vi "sub_Robot v1.vi"() -> ()   [LabVIEW 2017]
uses:
  <vilib>/Analysis/Matrix/Datatypes/RealMatrix.ctl
  Control/Force Torque Vector.ctl
  Control/State.ctl
  Control/Platform Vectors.ctl
  Control/Constants.ctl
  Control/Motor Position.ctl
  <vilib>/Analysis/baseanly.llb/A x Vector.vi
  <vilib>/DAQmx/read.llb/DAQmx Read (Analog 2D DBL NChan NSamp).vi
  <vilib>/Analysis/baseanly.llb/Mean (DBL).vi
  <vilib>/Analysis/baseanly.llb/Real A x B.vi
  <vilib>/Analysis/_algsub.llb/Vector Norm.vi
  <vilib>/Analysis/_algsub.llb/Real Vector Norm.vi
  <vilib>/Analysis/baseanly.llb/Outer Product.vi
  <vilib>/Analysis/baseanly.llb/Real Outer Product.vi
  <vilib>/robotics/Kinematics/Create Lie Group Matrix.vi
  <vilib>/Analysis/7linalg.llb/Create Special Real Matrix.vi
  <vilib>/Analysis/Matrix/Numeric/Multiply/Multiply.vi
  <vilib>/Analysis/Matrix/Numeric/Multiply/Multiply - RM,R.vi
  <vilib>/Analysis/Matrix/Numeric/Multiply/Multiply - R,RM.vi
  <vilib>/Analysis/Matrix/Numeric/Add/Add.vi
  <vilib>/Analysis/Matrix/Numeric/Add/Add - RM,RM.vi
  <vilib>/DAQmx/create/channels.llb/DAQmx Create Channel (AI-Voltage-Basic).vi
  <vilib>/DAQmx/configure/timing.llb/DAQmx Timing (Sample Clock).vi
  <vilib>/DAQmx/miscellaneous.llb/DAQmx Fill In Error Info.vi
  <vilib>/Analysis/3filter.llb/Butterworth Filter (DBL).vi
  <vilib>/Utility/inputDevices.llb/joystickAcquire.vi
  <vilib>/Analysis/NI_AALBase.lvlib
  <vilib>/robotics/Kinematics/NI_Kinematics.lvlib
  <vilib>/Analysis/NI_AALPro.lvlib
  <vilib>/Analysis/Matrix/NI_Matrix.lvlib
panel:
  in  "low cutoff freq: fl":dbl=0.1 format="%0.4f"
  in  "sampling freq: fs":dbl=100.0 format="%0.2f"
  in  "rate":dbl=1000.0 format="%#_13g"
  out "Motor Position":T1={"theta1"=1.8810837497796307, "theta2"=-0.7792215646198668, "theta3"=2.7030056815353944}
  in  "eta3":dbl=240.0
  in  "eta2":dbl=120.0
  in  "eta1":dbl
  out "dt":dbl=0.014741399998456473
  in  "gamma2":dbl=72.0
  in  "gamma1":dbl=90.0
  in  "alpha2":dbl=90.0
  in  "alpha1":dbl=90.0
  out "Constants":T2={"alpha1"=1.5707963267948966, "alpha2"=1.5707963267948966, "beta1"=0.9553166181245093, "beta2"=0.7460127831658564, "gamma1"=1.5707963267948966, "gamma2"=1.2566370614359172, "eta1"=0.0, "eta2"=2.0943951023931953, "eta3"=4.1887902047863905}
  out "Platform Vectors":T3={"v1"=[0.9518431395713998, -0.15246563731281282, 0.26598659193586577], "v2"=[0.43921969187034554, 0.8926089520236044, 0.10166278099993067], "v3"=[0.5741590303779587, 0.15523155866204005, -0.8038933828753619]}
  in  "radius":dbl=0.1
  in  "State":T4={"Inertia"=0.0, "Damping"=0.5, "RoM"=0.0}
  out "Waveform Chart":cluster{dbl, dbl, dbl}(graph)
  out "Force Torque Vector":T5
  in  "Calibration Matrix":T6=[[0.70287, 0.28046, -1.06379, -47.58271, -1.64459, 46.90249], [-0.12905, 55.12684, -1.23322, -27.09022, 0.94146, -27.44249], [69.23154, 1.17633, 67.18151, 0.05352, 69.14468, -0.82584], [0.02366, 0.38743, -1.10802, -0.19684, 1.1351, -0.20033], [1.26658, 0.02633, -0.60731, 0.32903, -0.6386, -0.32248], [0.02624, -0.70869, -0.00313, -0.69424, -0.02408, -0.68399]]
  in  "stop":bool
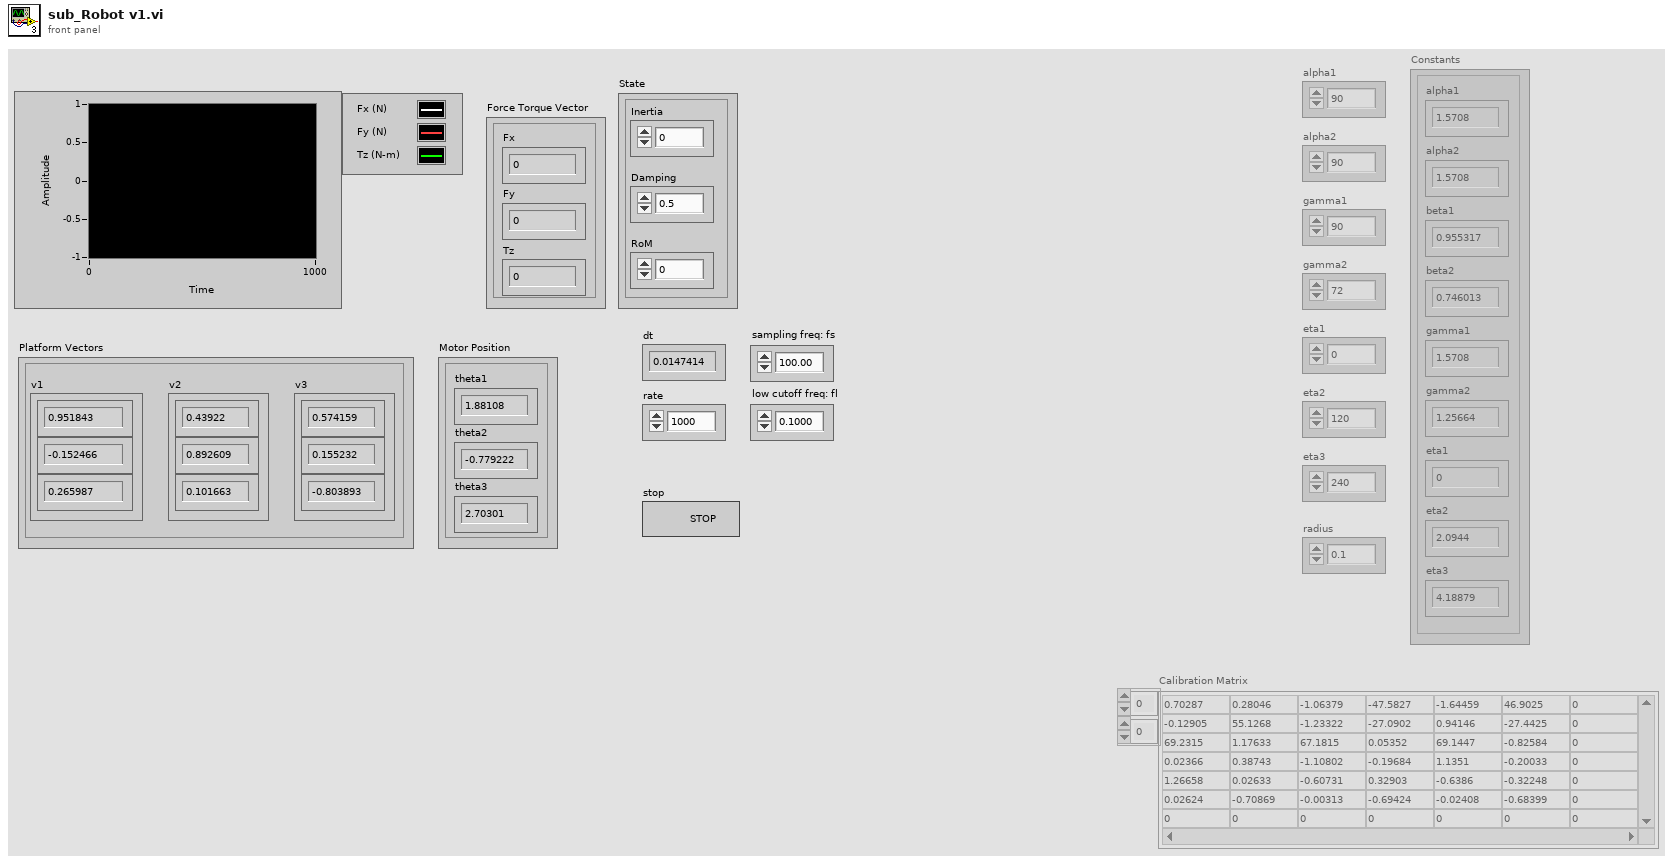
[diagram p1: front panel]
types:
  T1 = typedef "Motor Position.ctl" = cluster{"theta1":dbl, "theta2":dbl, "theta3":dbl}
  T2 = typedef "Constants.ctl" = cluster{"alpha1":dbl, "alpha2":dbl, "beta1":dbl, "beta2":dbl, "gamma1":dbl, "gamma2":dbl, "eta1":dbl, "eta2":dbl, "eta3":dbl}
  T3 = typedef "Platform Vectors.ctl" = cluster{"v1":dbl[], "v2":dbl[], "v3":dbl[]}
  T4 = typedef "State.ctl" = cluster{"Inertia":dbl, "Damping":dbl, "RoM":dbl}
  T5 = typedef "Force Torque Vector.ctl" = cluster{"Fx":dbl, "Fy":dbl, "Tz":dbl}
  T6 = typedef "NI_Matrix.lvlib/RealMatrix.ctl" = dbl[][]
  T7 = cluster{"X axis":i32, "Y axis":i32, "Z axis":i32, "X axis rotation":i32, "Y axis rotation":i32, "Z axis rotation":i32, "U axis":i32, "V axis":i32}
  T8 = cluster{"element":dbl, "element":dbl, "element":dbl}
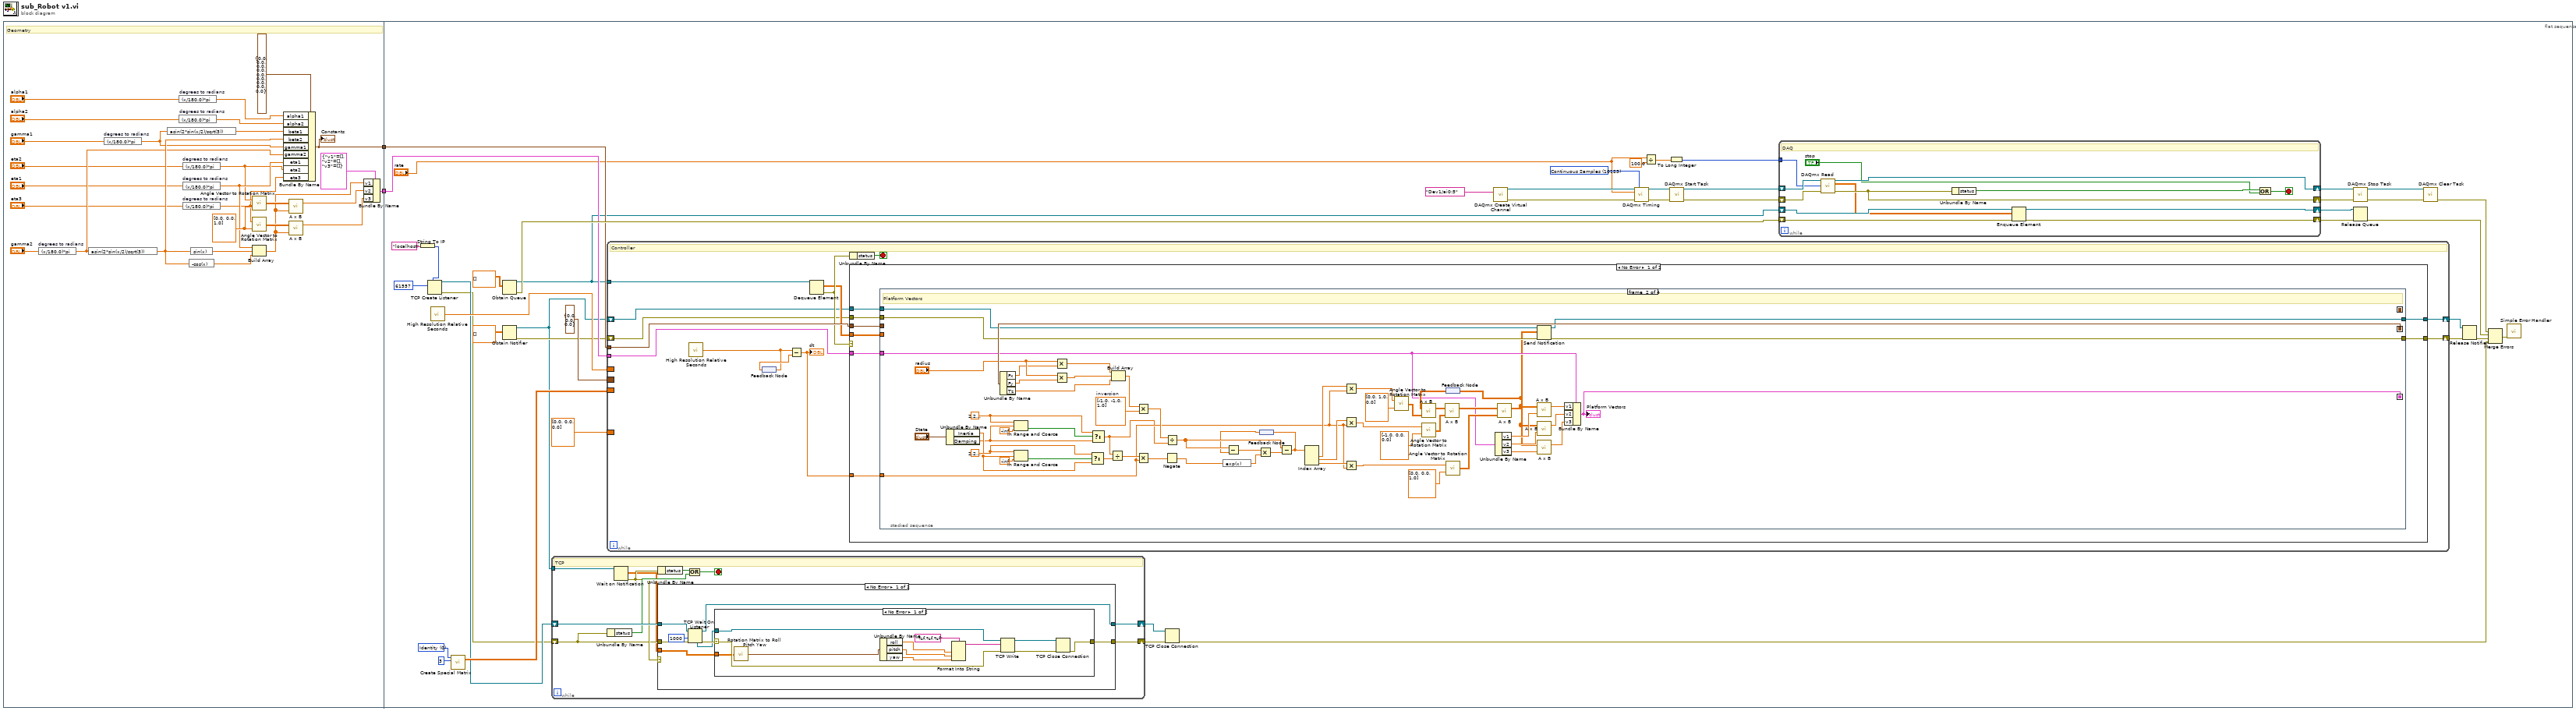
[diagram p0: block diagram]
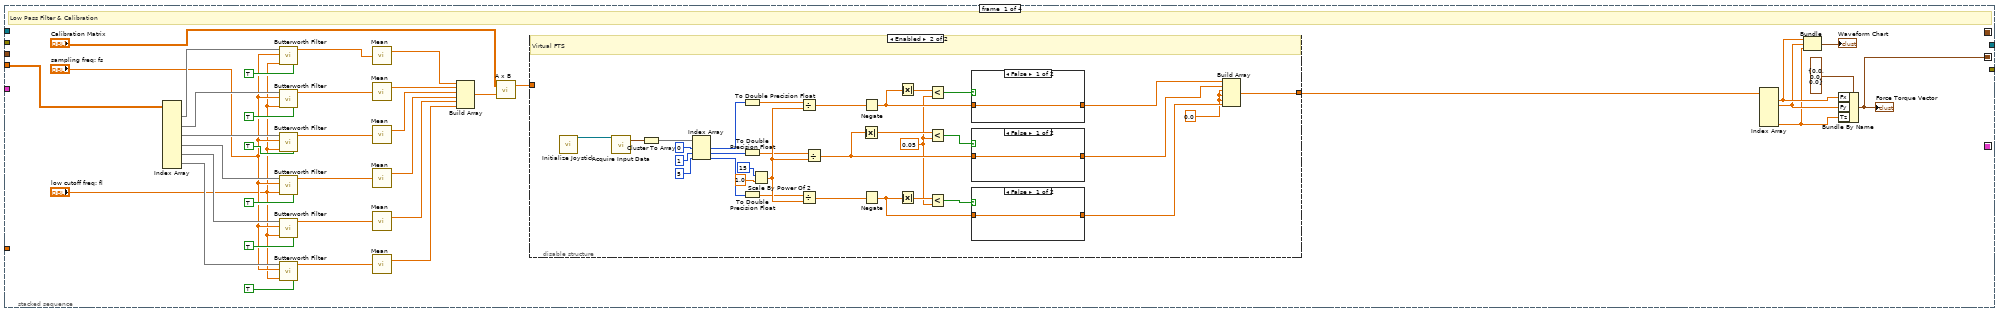
[diagram p4: hidden frame]
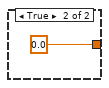
[diagram p6: hidden frame]
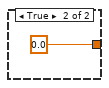
[diagram p7: hidden frame]
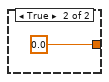
[diagram p8: hidden frame]
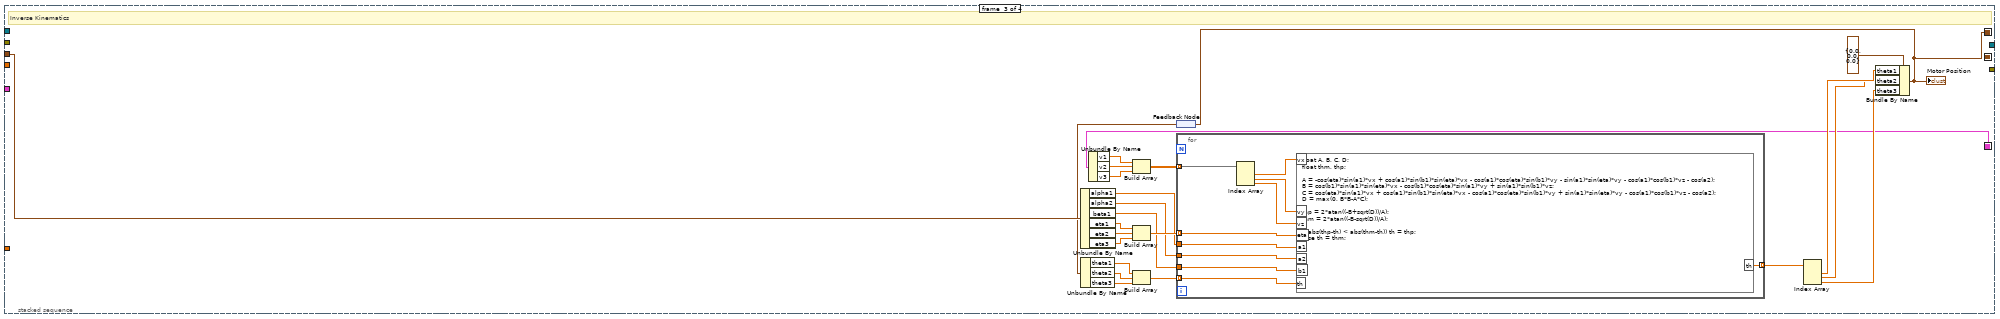
[diagram p9: hidden frame]
diagram:
  n1 = flat-sequence {
    tunnel: [w3] -> w2
    tunnel: [w5] -> w1
    tunnel: w2 -> [w54]
    tunnel: w1 -> [w53]
    frame #0 {
      w19 = dbl[] [0.0, 0.0, 1.0] ("vector")
      # "Geometry"
      n2 = expression code="(x/180.0)*pi" "degrees to radians"("gamma2") -> (w13:dbl)
      n3 = expression code="asin(2*sin(x/2)/sqrt(3))"(w13) -> (w15:dbl)
      n4 = expression code="(x/180.0)*pi" "degrees to radians"("gamma1") -> (w14:dbl)
      n5 = expression code="asin(2*sin(x/2)/sqrt(3))"(w14) -> (w26:dbl)
      n6 = expression code="(x/180.0)*pi" "degrees to radians"("alpha1") -> (w29:dbl)
      n7 = expression code="(x/180.0)*pi" "degrees to radians"("alpha2") -> (w27:dbl)
      n8 = expression code="(x/180.0)*pi" "degrees to radians"("eta2") -> (w8:dbl)
      n9 = expression code="(x/180.0)*pi" "degrees to radians"("eta1") -> (w9:dbl)
      n10 = expression code="(x/180.0)*pi" "degrees to radians"("eta3") -> (w7:dbl)
      n11 = expression code="-cos(x)"(w15) -> (w21:dbl)
      n12 = expression code="sin(x)"(w15) -> (w20:dbl)
      n13 = call <vilib>:"Angle Vector to Rotation Matrix.vi"("vector"=w19, "angle"=w8) -> ("rotation matrix"=w22:T6)
      n14 = call <vilib>:"Angle Vector to Rotation Matrix.vi"("vector"=w19, "angle"=w7) -> ("rotation matrix"=w23:T6)
      n15 = Build Array(w9, w20, w21) -> (w18:dbl[])
      n16 = Bundle By Name(cluster=T2 {"alpha1"=0.0, "alpha2"=0.0, "beta1"=0.0, "beta2"=0.0, "gamma1"=0.0, "gamma2"=0.0, "eta1"=0.0, "eta2"=0.0, "eta3"=0.0} ("Constants"), "alpha1"=w29, "alpha2"=w27, "beta1"=w26, "beta2"=w15, "gamma1"=w14, "gamma2"=w13, "eta1"=w9, "eta2"=w8, "eta3"=w7) -> (w5:T2)
      "Constants" <- w5
      n17 = call-poly <vilib>:"A x B.vi"("Vector"=w18, "A"=w22) -> ("A x Vector"=w17:dbl[])  [unwired: 1 out]
      n18 = call-poly <vilib>:"A x B.vi"("Vector"=w18, "A"=w23) -> ("A x Vector"=w16:dbl[])  [unwired: 1 out]
      n19 = Bundle By Name(cluster=T3 {"v1"=[], "v2"=[], "v3"=[]} ("Platform Vectors"), "v1"=w18, "v2"=w17, "v3"=w16) -> (w3:T3)
    }
    frame #1 {
      w57 = 0 items=["Identity", "Diagonal", "Toeplitz", "Vandermonde", "Companion", "Hankel", "Hadamard", "Wilkinson", "Hilbert", "Inverse Hilbert", "Rosser", "Pascal"] ("matrix type")
      w65 = 10123 items=["Finite Samples"=10178, "Continuous Samples"=10123, "Hardware Timed Single Point"=12522] ("sample mode")
      n20 = String To IP(1:"localhost" ("name")) -> (0:w33:u32)
      n21 = TCP Create Listener(7:w33, 10:u16 61557 ("port")) -> (0:w31:errorcluster, 3:w32:refnum<k5>)  [unwired: 3 in, 1 out]
      n22 = call <vilib>:"High Resolution Relative Seconds.vi"() -> ("relative seconds"=w46:dbl)
      n23 = call-poly <vilib>:"Create Special Matrix.vi"("matrix type"=w57, "matrix size"=3) -> ("Special Matrix"=w55:T6)  [unwired: 3 in, 1 out]
      n24 = Obtain Queue(element data type=dbl[][] [] ("data")) -> (queue out=w51:refnum<queue>, error out=w64:errorcluster)  [unwired: 4 in, 1 out]
      n25 = Obtain Notifier(notification data type=T6 [] ("A x B")) -> (notifier out=w40:refnum<notifier>, error out=w44:errorcluster)  [unwired: 3 in, 1 out]
      n26 = while {
        tunnel: w40 -> [w86]
        shift-right: [w84] -> w37
        shift-left: w31 -> [w79]
        shift-right: [w85] -> w38
        shift-left: w32 -> [w83]
        stop <- w78 stop-if-true
        # "TCP"
        n27 = Unbundle By Name(w79) -> ("status"=w81:bool)
        n28 = Wait on Notification(notifier=w86) -> (notification=w77:T6, error out=w80:errorcluster)  [unwired: 3 in, 2 out]
        n29 = Unbundle By Name(w80) -> ("status"=w82:bool)
        n30 = case shown="No Error" w80 {
          tunnel: w79 -> [w93 w108]
          tunnel: [w92 w109] -> w85
          tunnel: [w90 w108] -> w84
          tunnel: w83 -> [w89 w109]
          tunnel: w77 -> [w88 _]
          frame No Error {
            n31 = TCP Wait On Listener(8:w93, 9:1000 ("timeout ms (wait forever: -1)"), 11:w89) -> (0:w94:errorcluster, 3:w92:refnum<k5>, 4:w91:refnum<k5>)  [unwired: 1 in, 2 out]
            n32 = case shown="No Error" w94 {
              selector: w94 -> [w102 w107]
              tunnel: w91 -> [w105 _]
              tunnel: [w103 w107] -> w90
              tunnel: w88 -> [w96 _]
              frame No Error {
                n33 = call <vilib>:"Rotation Matrix to Roll Pitch Yaw.vi"("rotation matrix"=w96) -> ("angles"=w98:cluster{"roll":dbl, "pitch":dbl, "yaw":dbl})
                n34 = Unbundle By Name(w98) -> ("roll"=w99:dbl, "pitch"=w100:dbl, "yaw"=w101:dbl)
                n35 = Format Into String(format string="%f,%f,%f", w99, w100, w101) -> (resulting string=w95:string)  [unwired: 2 in, 1 out]
                n36 = TCP Write(connection ID=w105, data in=w95, error in (no error)=w102) -> (connection ID out=w106:refnum<k5>, error out=w104:errorcluster)  [unwired: 1 in, 1 out]
                n37 = TCP Close Connection(connection ID=w106, error in (no error)=w104) -> (error out=w103:errorcluster)  [unwired: 1 in, 1 out]
              }
              frame Error {
              }
            }
          }
          frame Error {
          }
        }
        n38 = Compound Arithmetic op=OR(w82, w81) -> (w78:bool)
      }
      n39 = while {
        tunnel: w51 -> [w122]
        border: dbl[] [0.0, 0.0, 0.0] -> [_]
        border: w55 -> [_]
        tunnel: w53 -> [w120]
        border: T1 {"theta1"=0.0, "theta2"=0.0, "theta3"=0.0} ("Motor Position") -> [_]
        border: w46 -> [_]
        tunnel: w54 -> [w121]
        shift-right: [w113] -> w43
        shift-left: w40 -> [w114]
        shift-right: [w111] -> w42
        shift-left: w44 -> [w112]
        stop <- w110 stop-if-true
        # "Controller"
        n40 = call <vilib>:"High Resolution Relative Seconds.vi"() -> ("relative seconds"=w116:dbl)
        n41 = feedback-in #1(w116) -> ()
        n42 = feedback #1() -> (w117:dbl)
        n43 = Subtract(x=w116, y=w117) -> (x-y=w115:dbl)
        "dt" <- w115
        n44 = Dequeue Element(queue=w122) -> (element=w118:dbl[][], error out=w119:errorcluster)  [unwired: 2 in, 2 out]
        n45 = Unbundle By Name(w119) -> ("status"=w110:bool)
        n46 = case shown="No Error" w119 {
          tunnel: w121 -> [w130 _]
          tunnel: w120 -> [w129 _]
          tunnel: w118 -> [w128 _]
          tunnel: w115 -> [w127 _]
          tunnel: w114 -> [w126 w301]
          tunnel: [w123 w301] -> w113
          tunnel: w112 -> [w125 w300]
          tunnel: [w124 w300] -> w111
          frame No Error {
            n47 = stacked-sequence {
              seq-local: [w165 _ _ _] -> [_ w244 _ _]
              seq-local: [_ w227 _ _] -> [_ _ w268 _]
              seq-local: [_ _ w266 _] -> [_ _ _ _]
              tunnel: w130 -> [_ w231 _ _]
              tunnel: w129 -> [_ _ w285 _]
              tunnel: w127 -> [_ w226 _ _]
              tunnel: w128 -> [w137 _ _ _]
              tunnel: w126 -> [_ w211 _ _]
              tunnel: w125 -> [_ w210 _ _]
              tunnel: [_ w209 _ _] -> w124
              tunnel: [_ w208 _ _] -> w123
              frame #0 {
                # "Low Pass Filter & Calibration"
                n48 = Index Array(array=w137) -> (element #1=w148:dbl[], element #2=w147:dbl[], element #3=w146:dbl[], element #4=w145:dbl[], element #5=w144:dbl[], element #6=w143:dbl[])  [unwired: 12 in]
                n49 = call-poly <vilib>:"Butterworth Filter.vi"("init/cont (init:F)"=TRUE, "low cutoff freq: fl"="low cutoff freq: fl", "sampling freq: fs"="sampling freq: fs", "X"=w148) -> ("Filtered X"=w149:dbl[])  [unwired: 4 in, 1 out]
                n50 = call-poly <vilib>:"Butterworth Filter.vi"("init/cont (init:F)"=TRUE, "low cutoff freq: fl"="low cutoff freq: fl", "sampling freq: fs"="sampling freq: fs", "X"=w147) -> ("Filtered X"=w151:dbl[])  [unwired: 4 in, 1 out]
                n51 = call-poly <vilib>:"Butterworth Filter.vi"("init/cont (init:F)"=TRUE, "low cutoff freq: fl"="low cutoff freq: fl", "sampling freq: fs"="sampling freq: fs", "X"=w146) -> ("Filtered X"=w153:dbl[])  [unwired: 4 in, 1 out]
                n52 = call-poly <vilib>:"Butterworth Filter.vi"("init/cont (init:F)"=TRUE, "low cutoff freq: fl"="low cutoff freq: fl", "sampling freq: fs"="sampling freq: fs", "X"=w145) -> ("Filtered X"=w154:dbl[])  [unwired: 4 in, 1 out]
                n53 = call-poly <vilib>:"Butterworth Filter.vi"("init/cont (init:F)"=TRUE, "low cutoff freq: fl"="low cutoff freq: fl", "sampling freq: fs"="sampling freq: fs", "X"=w144) -> ("Filtered X"=w155:dbl[])  [unwired: 4 in, 1 out]
                n54 = call-poly <vilib>:"Butterworth Filter.vi"("init/cont (init:F)"=TRUE, "low cutoff freq: fl"="low cutoff freq: fl", "sampling freq: fs"="sampling freq: fs", "X"=w143) -> ("Filtered X"=w159:dbl[])  [unwired: 4 in, 1 out]
                n55 = call-poly <vilib>:"Mean.vi"("X"=w149) -> ("mean"=w150:dbl)  [unwired: 1 out]
                n56 = call-poly <vilib>:"Mean.vi"("X"=w151) -> ("mean"=w152:dbl)  [unwired: 1 out]
                n57 = call-poly <vilib>:"Mean.vi"("X"=w153) -> ("mean"=w156:dbl)  [unwired: 1 out]
                n58 = call-poly <vilib>:"Mean.vi"("X"=w154) -> ("mean"=w157:dbl)  [unwired: 1 out]
                n59 = call-poly <vilib>:"Mean.vi"("X"=w155) -> ("mean"=w158:dbl)  [unwired: 1 out]
                n60 = call-poly <vilib>:"Mean.vi"("X"=w159) -> ("mean"=w160:dbl)  [unwired: 1 out]
                n61 = Build Array(w150, w152, w156, w157, w158, w160) -> (w135:dbl[])
                n62 = call-poly <vilib>:"A x B.vi"("Vector"=w135, "A"="Calibration Matrix") -> ("A x Vector"=w131:dbl[])  [unwired: 1 out]
                n63 = disable-structure shown="Enabled" {
                  disable-tunnel: [w168 w176] -> w132
                  disable-tunnel: w131 -> [w168 _]
                  frame Disabled {
                  }
                  frame Enabled {
                    w175 = 0.0 ("element")
                    w180 = 0.05 ("y")
                    # "Virtual FTS"
                    n64 = call <vilib>:"Initialize Joystick.vi"() -> ("device ID"=w193:refnum<k1>)  [unwired: 10 in, 1 out]
                    n65 = call-poly <vilib>:"Acquire Input Data.vi"("device ID"=w193) -> ("axis info"=w200:T7)  [unwired: 14 in, 4 out]
                    n66 = Cluster To Array(cluster=w200) -> (array=w196:i32[])
                    n67 = Index Array(array=w196, index #1=0 ("index"), index #2=1 ("index"), index #3=5 ("index")) -> (element #1=w174:i32, element #2=w172:i32, element #3=w170:i32)
                    n68 = To Double Precision Float(number=w174) -> (double precision float=w173:dbl)
                    n69 = To Double Precision Float(number=w172) -> (double precision float=w171:dbl)
                    n70 = To Double Precision Float(number=w170) -> (double precision float=w169:dbl)
                    n71 = Scale By Power Of 2(n=i16 15, x=1.0) -> (x*2^n=w188:dbl)
                    n72 = Divide(x=w173, y=w188) -> (x/y=w192:dbl)
                    n73 = Divide(x=w169, y=w188) -> (x/y=w181:dbl)
                    n74 = Divide(x=w171, y=w188) -> (x/y=w183:dbl)
                    n75 = Absolute Value(x=w183) -> (abs(x)=w190:dbl)
                    n76 = Negate(x=w192) -> (-x=w184:dbl)
                    n77 = Negate(x=w181) -> (-x=w182:dbl)
                    n78 = Absolute Value(x=w184) -> (abs(x)=w191:dbl)
                    n79 = Absolute Value(x=w182) -> (abs(x)=w189:dbl)
                    n80 = Less?(x=w191, y=w180) -> (x < y?=w187:bool)
                    n81 = Less?(x=w190, y=w180) -> (x < y?=w186:bool)
                    n82 = Less?(x=w189, y=w180) -> (x < y?=w185:bool)
                    n83 = case shown="False" w187 {
                      tunnel: [w205 0.0] -> w179
                      tunnel: w184 -> [w205 _]
                      frame False {
                      }
                      frame True {
                      }
                    }
                    n84 = case shown="False" w186 {
                      tunnel: [w203 0.0] -> w178
                      tunnel: w183 -> [w203 _]
                      frame False {
                      }
                      frame True {
                      }
                    }
                    n85 = case shown="False" w185 {
                      tunnel: [w201 0.0] -> w177
                      tunnel: w182 -> [w201 _]
                      frame False {
                      }
                      frame True {
                      }
                    }
                    n86 = Build Array(w179, w178, w175, w175, w175, w177) -> (w176:dbl[])
                  }
                }
                n87 = Index Array(array=w132) -> (element #1=w164:dbl, element #2=w163:dbl, element #6=w162:dbl)  [unwired: 6 in, 3 out]
                n88 = Bundle("element"=w164, "element"=w163, "element"=w162) -> (→"Waveform Chart":T8)  [unwired: 1 in]
                n89 = Bundle By Name(cluster=T5 {"Fx"=0.0, "Fy"=0.0, "Tz"=0.0} ("Force Torque Vector"), "Fx"=w164, "Fy"=w163, "Tz"=w162) -> (w165:T5)
                "Force Torque Vector" <- w165
              }
              frame #1 {
                w216 = 2.220446049250313e-16
                w219 = 2.220446049250313e-16
                w229 = dbl[] [-1.0, -1.0, 1.0]  # inversion
                # "Platform Vectors"
                n90 = Unbundle By Name("State") -> ("Inertia"=w218:dbl, "Damping"=w213:dbl)
                n91 = Unbundle By Name(w244) -> ("Fx"=w242:dbl, "Fy"=w241:dbl, "Tz"=w238:dbl)
                n92 = In Range and Coerce(upper limit=w216, x=w213, lower limit=-inf) -> (In Range?=w215:bool)  [unwired: 1 out]
                n93 = In Range and Coerce(upper limit=w219, x=w218, lower limit=-inf) -> (In Range?=w220:bool)  [unwired: 1 out]
                n94 = Multiply(x="radius", y=w242) -> (x*y=w240:dbl)
                n95 = Multiply(x="radius", y=w241) -> (x*y=w239:dbl)
                n96 = Select(t=w219, s=w220, f=w218) -> (s? t:f=w217:dbl)
                n97 = Select(t=w216, s=w215, f=w213) -> (s? t:f=w212:dbl)
                n98 = Divide(x=w212, y=w217) -> (x/y=w255:dbl)
                n99 = Build Array(w240, w239, w238) -> (w230:dbl[])
                n100 = Multiply(x=w230, y=w229) -> (x*y=w228:dbl[])
                n101 = Multiply(x=w255, y=w226) -> (x*y=w254:dbl)
                n102 = Negate(x=w254) -> (-x=w253:dbl)
                n103 = Divide(x=w228, y=w212) -> (x/y=w250:dbl[])
                n104 = expression code="exp(x)"(w253) -> (w251:dbl)
                n105 = feedback #2() -> (w236:dbl[])
                n106 = Subtract(x=w250, y=w236) -> (x-y=w252:dbl[])
                n107 = Multiply(x=w252, y=w251) -> (x*y=w249:dbl[])
                n108 = Subtract(x=w250, y=w249) -> (x-y=w237:dbl[])
                n109 = feedback-in #2(w237) -> ()
                n110 = Index Array(array=w237) -> (element #1=w247:dbl, element #2=w246:dbl, element #3=w248:dbl)  [unwired: 3 in]
                n111 = Multiply(x=w247, y=w226) -> (x*y=w265:dbl)
                n112 = Multiply(x=w246, y=w226) -> (x*y=w264:dbl)
                n113 = Multiply(x=w248, y=w226) -> (x*y=w225:dbl)
                n114 = call <vilib>:"Angle Vector to Rotation Matrix.vi"("vector"=dbl[] [0.0, 1.0, 0.0], "angle"=w265) -> ("rotation matrix"=w260:T6)
                n115 = call <vilib>:"Angle Vector to Rotation Matrix.vi"("vector"=dbl[] [-1.0, 0.0, 0.0], "angle"=w264) -> ("rotation matrix"=w258:T6)
                n116 = feedback #3() -> (w235:T6)
                n117 = call-poly <vilib>:"A x B.vi"("B"=w260, "A"=w235) -> ("A x B"=w259:T6)  [unwired: 1 out]
                n118 = call-poly <vilib>:"A x B.vi"("B"=w258, "A"=w259) -> ("A x B"=w257:T6)  [unwired: 1 out]
                n119 = call <vilib>:"Angle Vector to Rotation Matrix.vi"("vector"=dbl[] [0.0, 0.0, 1.0], "angle"=w225) -> ("rotation matrix"=w256:T6)
                n120 = Unbundle By Name(w231) -> ("v1"=w234:dbl[], "v2"=w233:dbl[], "v3"=w232:dbl[])
                n121 = call-poly <vilib>:"A x B.vi"("B"=w256, "A"=w257) -> ("A x B"=w207:T6)  [unwired: 1 out]
                n122 = feedback-in #3(w207) -> ()
                n123 = Send Notification(notification=w207, notifier=w211, error in (no error)=w210) -> (notifier out=w208:refnum<notifier>, error out=w209:errorcluster)
                n124 = call-poly <vilib>:"A x B.vi"("Vector"=w234, "A"=w207) -> ("A x Vector"=w224:dbl[])  [unwired: 1 out]
                n125 = call-poly <vilib>:"A x B.vi"("Vector"=w233, "A"=w207) -> ("A x Vector"=w223:dbl[])  [unwired: 1 out]
                n126 = call-poly <vilib>:"A x B.vi"("Vector"=w232, "A"=w207) -> ("A x Vector"=w222:dbl[])  [unwired: 1 out]
                n127 = Bundle By Name(cluster=w231, "v1"=w224, "v2"=w223, "v3"=w222) -> (w227:T3)
                "Platform Vectors" <- w227
              }
              frame #2 {
                # "Inverse Kinematics"
                n128 = Unbundle By Name(w285) -> ("alpha1"=w280:dbl, "alpha2"=w279:dbl, "beta1"=w278:dbl, "eta1"=w284:dbl, "eta2"=w283:dbl, "eta3"=w282:dbl)
                n129 = Unbundle By Name(w268) -> ("v1"=w289:dbl[], "v2"=w288:dbl[], "v3"=w287:dbl[])
                n130 = Build Array(w289, w288, w287) -> (w286:dbl[][])
                n131 = Build Array(w284, w283, w282) -> (w281:dbl[])
                n132 = feedback #4() -> (w273:T1)
                n133 = Unbundle By Name(w273) -> ("theta1"=w272:dbl, "theta2"=w271:dbl, "theta3"=w270:dbl)
                n134 = Build Array(w272, w271, w270) -> (w269:dbl[])
                n135 = for {
                  tunnel: w286 -> [w299] mode=indexing
                  tunnel: w281 -> [w295] mode=indexing
                  tunnel: w280 -> [w294]
                  tunnel: w279 -> [w293]
                  tunnel: w278 -> [w292]
                  tunnel: [w291] -> w277 mode=indexing
                  tunnel: w269 -> [w290] mode=indexing
                  n136 = Index Array(array=w299) -> (element #1=w298:dbl, element #2=w297:dbl, element #3=w296:dbl)  [unwired: 3 in]
                  n137 = formula code="float A, B, C, D;\nfloat thm, thp;\n\nA = -cos(eta)*sin(a1)*vx + cos(a1)*sin(b1)*sin(eta)*vx - cos(a1)*cos(eta)*sin(b1)*vy - sin(a1)*sin(eta)*vy - cos(a1)*cos(b1)*vz - cos(a2);\nB = cos(b1)*sin(a1)*sin(eta)*vx - cos(b1)*cos(eta)*sin(a1)*vy + sin(a1)*sin(b1)*vz;\nC = cos(eta)*sin(a1)*vx + cos(a1)*sin(b1)*sin(eta)*vx - cos(a1)*cos(eta)*sin(b1)*vy + sin(a1)*sin(eta)*vy - cos(a1)*cos(b1)*vz - cos(a2);\nD = max(0, B*B-A*C);\n\nthp = 2*atan((-B+sqrt(D))/A); \nthm = 2*atan((-B-sqrt(D))/A); \n\nif(abs(thp-th) < abs(thm-th)) th = thp;\nelse th = thm;"("vx"=w298, "vy"=w297, "vz"=w296, "eta"=w295, "a1"=w294, "b1"=w292, "a2"=w293, "th"=w290) -> ("th"=w291:dbl)
                }
                n138 = Index Array(array=w277) -> (element #1=w276:dbl, element #2=w275:dbl, element #3=w274:dbl)  [unwired: 3 in]
                n139 = Bundle By Name(cluster=T1 {"theta1"=0.0, "theta2"=0.0, "theta3"=0.0} ("Motor Position"), "theta1"=w276, "theta2"=w275, "theta3"=w274) -> (w266:T1)
                "Motor Position" <- w266
                n140 = feedback-in #4(w266) -> ()
              }
              frame #3 {
                # "myRIO"
              }
            }
          }
          frame Error {
          }
        }
      }
      n141 = TCP Close Connection(connection ID=w38, error in (no error)=w37) -> (error out=w36:errorcluster)  [unwired: 1 in, 1 out]
      n142 = call-poly <vilib>:"DAQmx Create Virtual Channel.vi"("physical channels"=tag "Dev1/ai0:5") -> ("task out"=w75:refnum<k21>, "error out"=w74:errorcluster)  [unwired: 13 in]
      n143 = call-poly <vilib>:"DAQmx Timing.vi"("task/channels in"=w75, "sample mode"=w65, "rate"="rate", "error in"=w74) -> ("task out"=w72:refnum<k21>, "error out"=w73:errorcluster)  [unwired: 10 in]
      n144 = Divide(x="rate", y=100.0) -> (x/y=w45:dbl)
      n145 = To Long Integer(number=w45) -> (32bit integer=w48:i32)
      n146 = call <vilib>:"DAQmx Start Task.vi"("task/channels in"=w72, "error in"=w73) -> ("task out"=w71:refnum<k21>, "error out"=w68:errorcluster)  [unwired: 12 in]
      n147 = while {
        shift-right: [w309] -> w61
        shift-left: w51 -> [w310]
        shift-right: [w306] -> w60
        shift-left: w64 -> [w308]
        shift-right: [w313] -> w70
        shift-left: w71 -> [w314]
        shift-right: [w311] -> w67
        shift-left: w68 -> [w312]
        tunnel: w48 -> [w302]
        stop <- w305 stop-if-true
        # "DAQ"
        n148 = call-poly <vilib>:"DAQmx Read.vi"("task/channels in"=w314, "number of samples per channel"=w302, "error in"=w312) -> ("task out"=w313:refnum<k21>, "data"=w303:dbl[][], "error out"=w311:errorcluster)  [unwired: 10 in]
        n149 = Unbundle By Name(w311) -> ("status"=w307:bool)
        n150 = Enqueue Element(queue=w310, element=w303, error in (no error)=w308) -> (queue out=w309:refnum<queue>, error out=w306:errorcluster)  [unwired: 1 in, 1 out]
        n151 = Compound Arithmetic op=OR(w307, "stop") -> (w305:bool)
      }
      n152 = call <vilib>:"DAQmx Stop Task.vi"("task/channels in"=w70, "error in"=w67) -> ("task out"=w69:refnum<k21>, "error out"=w66:errorcluster)  [unwired: 12 in]
      n153 = Release Queue(queue=w61, error in (no error)=w60) -> (error out=w59:errorcluster)  [unwired: 1 in, 2 out]
      n154 = call <vilib>:"DAQmx Clear Task.vi"("task in"=w69, "error in"=w66) -> ("error out"=w62:errorcluster)  [unwired: 13 in]
      n155 = Release Notifier(notifier=w43, error in (no error)=w42) -> (error out=w41:errorcluster)  [unwired: 1 in, 2 out]
      n156 = Merge Errors(w62, w59, w41, w36) -> (w63:errorcluster)
      n157 = call <vilib>:"Simple Error Handler.vi"("error in (no error)"=w63) -> ()  [unwired: 4 in, 5 out]
    }
  }
